vi "Parse Cave System.vi"(11 "Input":string) -> (3 "Cave System":T1)   [LabVIEW 2020]
uses:
  Cave System.ctl
  Cave.ctl
  <vilib>/regexp/Match Regular Expression.xnode
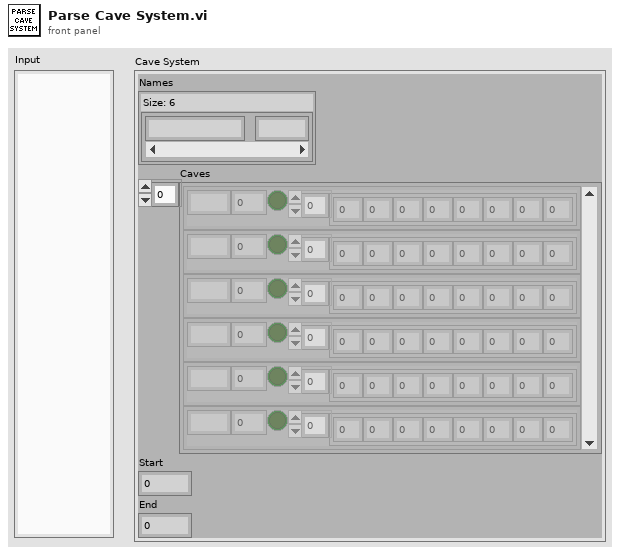
[diagram p1: front panel]
types:
  T1 = typedef "Cave System.ctl" = cluster{"Names":map{string, i32}, "Caves":T2[], "Start":i32, "End":i32}
  T2 = typedef "Cave.ctl" = cluster{"Name":string, "Index":i32, "Big":bool, "Links":i32[]}
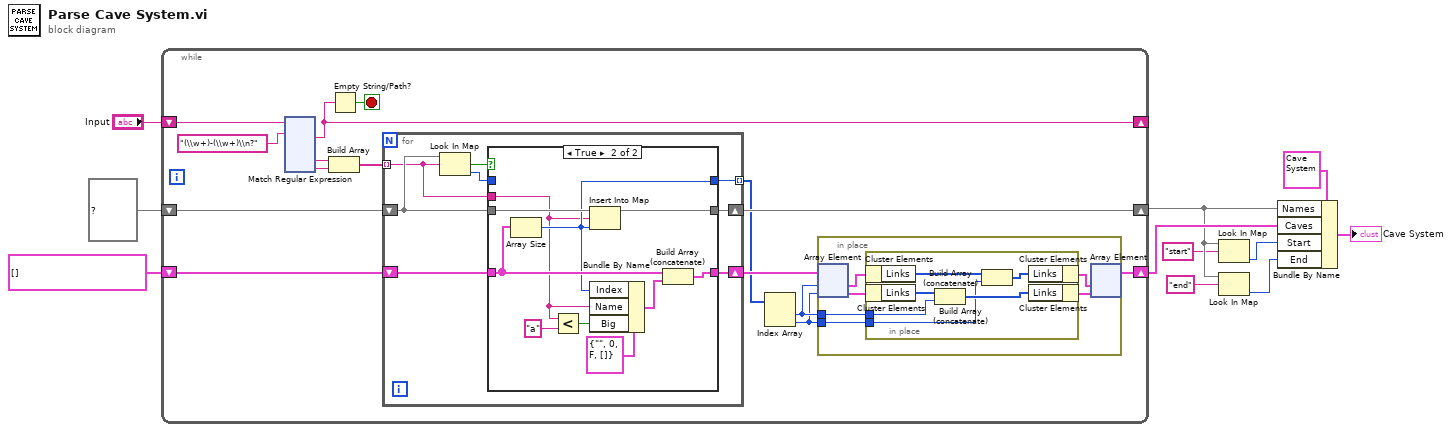
[diagram p0: block diagram]
diagram:
  n1 = while {
    shift-right: [w24] -> _
    shift-left: "Input" -> [w26]
    shift-right: [w17] -> w6
    shift-left: map{string, i32} {} ("map") -> [w19]
    shift-right: [w14] -> w7
    shift-left: T2[] [] -> [w18]
    stop <- w23 stop-if-true
    n2 = xnode "Match Regular Expression"("input string"=w26, "regular expression"="(\\w+)-(\\w+)\\n?") -> ("after match"=w24:string, "submatch 1"=w22:string, "submatch 2"=w21:string)  [unwired: 4 in, 4 out]
    n3 = Build Array(w22, w21) -> (w20:string[])
    n4 = Empty String/Path?(string/path=w24) -> (empty?=w23:bool)
    n5 = for {
      tunnel: w20 -> [w42] mode=indexing
      shift-right: [w40] -> w17
      shift-left: w19 -> [w46]
      shift-right: [w41] -> w16
      shift-left: w18 -> [w45]
      tunnel: [w39] -> w15 mode=indexing
      n6 = Look In Map(map=w46, key=w42) -> (key not found?=w44:bool, value=w43:i32)  [unwired: 1 in]
      n7 = case shown="True" w44 {
        tunnel: w46 -> [w48 w59]
        tunnel: w45 -> [w49 w55]
        tunnel: w43 -> [w47 _]
        tunnel: w42 -> [_ w50]
        tunnel: [w49 w51] -> w41
        tunnel: [w48 w52] -> w40
        tunnel: [w47 w53] -> w39
        frame False {
        }
        frame True {
          n8 = Array Size(array=w55) -> (size(s)=w53:i32)
          n9 = Less?(x=w50, y="a") -> (x < y?=w57:bool)
          n10 = Insert Into Map(map in=w59, key=w50, value=w53) -> (map out=w52:map{string, i32})  [unwired: 2 out]
          n11 = Bundle By Name(cluster=T2 {"Name"="", "Index"=0, "Big"=FALSE, "Links"=[]} ("Cave"), "Index"=w53, "Name"=w50, "Big"=w57) -> (w54:T2)
          n12 = Build Array (concatenate)(w55, w54) -> (w51:T2[])
        }
      }
    }
    n13 = Index Array(array=w15) -> (element #1=w13:i32, element #2=w12:i32)  [unwired: 2 in]
    n14 = in-place {
      in-place-border: w13 -> [w30]
      in-place-border: w12 -> [w29]
      n15 = in-place-array #1(w16, w13, w12) -> (w32:T2, w31:T2)
      n16 = in-place {
        in-place-border: w30 -> [w37]
        in-place-border: w29 -> [w34]
        n17 = in-place-cluster #2(w32) -> ("Links"=w35:i32[])
        n18 = in-place-cluster #3(w31) -> ("Links"=w38:i32[])
        n19 = Build Array (concatenate)(w38, w37) -> (w36:i32[])
        n20 = Build Array (concatenate)(w35, w34) -> (w33:i32[])
        n21 = in-place-cluster #2("Links"=w33) -> (w28:T2)
        n22 = in-place-cluster #3("Links"=w36) -> (w27:T2)
      }
      n23 = in-place-array #1(w28, w27) -> (w14:T2[])  [unwired: 2 out]
    }
  }
  n24 = Look In Map(map=w6, key="start" ("y")) -> (value=w4:i32)  [unwired: 1 in, 1 out]
  n25 = Look In Map(map=w6, key="end" ("y")) -> (value=w2:i32)  [unwired: 1 in, 1 out]
  n26 = Bundle By Name(cluster=T1 {"Names"={}, "Caves"=[], "Start"=0, "End"=0} ("Cave System"), "Names"=w6, "Caves"=w7, "Start"=w4, "End"=w2) -> (→"Cave System":T1)
